vi "vew -- set temperature PID.vi"() -> ()   [LabVIEW 2012]
uses:
  ctl -- name dispatcher -- action.ctl
  tale of three indices.vi
  linear interpolation - real.vi
  line -- complex.vi
  Q -- check range -- i -- integer.vi
  command stack.vi
  tale of three indices -- check state.vi
  Q - not nan -- integer.vi
panel:
  out "df out":dbl
  out "Numeric":i32
  out "Plot: slope 2":cluster{dbl[], dbl[]}[](graph)=[{[], []}, {[10.0, 79.9, 149.8, 219.70000000000002, 289.6, 359.5, 429.40000000000003, 499.30000000000007, 569.2, 639.1, 709.0, 778.9000000000001, 848.8000000000001, 918.7, 988.6000000000001, 1058.5, 1128.4, 1198.3000000000002, 1268.2, 1338.1000000000001, 1408.0, 1477.9, 1547.8000000000002, 1617.7, 1687.6000000000001, 1757.5000000000002, 1827.4, 1897.3000000000002, 1967.2000000000003, 2037.1000000000001, 2107.0, 2176.9, 2246.8, 2316.7000000000003, 2386.6000000000004, 2456.5, 2526.4, 2596.3, 2666.2000000000003, 2736.1000000000004, 2806.0, 2875.9, 2945.8, 3015.7000000000003, 3085.6000000000004, 3155.5000000000005, 3225.4, 3295.3, 3365.2000000000003, 3435.1000000000004, 3505.0000000000005, 3574.9, 3644.8, 3714.7000000000003, 3784.6000000000004, 3854.5000000000005, 3924.4000000000005, 3994.3, 4064.2000000000003, 4134.1, 4204.0, 4273.900000000001, 4343.8, 4413.700000000001, 4483.6, 4553.5, 4623.400000000001, 4693.3, 4763.200000000001, 4833.1, 4903.0, 4972.900000000001, 5042.8, 5112.700000000001, 5182.6, 5252.5, 5322.400000000001, 5392.3, 5462.200000000001, 5532.1, 5602.0, 5671.900000000001, 5741.8, 5811.700000000001, 5881.6, 5951.500000000001, 6021.400000000001, 6091.3, 6161.200000000001, 6231.1, 6301.000000000001, 6370.900000000001, 6440.8, 6510.700000000001, 6580.6, 6650.500000000001, 6720.400000000001, 6790.3, 6860.200000000001, 6930.1], [1.0, 1.0, 1.0, 1.0, 1.0, 1.0, 1.0, 1.0, 1.0, 1.0, 1.0, 1.0, 1.0, 1.0, 1.0, 1.0, 1.0, 1.0, 1.0, 1.0, 1.0, 1.0, 1.0, 1.0, 1.0, 1.0, 1.0, 1.0, 1.0, 1.0, 1.0, 1.0, 1.0, 1.0, 1.0, 1.0, 1.0, 1.0, 1.0, 1.0, 1.0, 1.0, 1.0, 1.0, 1.0, 1.0, 1.0, 1.0, 1.0, 1.0, 1.0, 1.0, 1.0, 1.0, 1.0, 1.0, 1.0, 1.0, 1.0, 1.0, 1.0, 1.0, 1.0, 1.0, 1.0, 1.0, 1.0, 1.0, 1.0, 1.0, 1.0, 1.0, 1.0, 1.0, 1.0, 1.0, 1.0, 1.0, 1.0, 1.0, 1.0, 1.0, 1.0, 1.0, 1.0, 1.0, 1.0, 1.0, 1.0, 1.0, 1.0, 1.0, 1.0, 1.0, 1.0, 1.0, 1.0, 1.0, 1.0, 1.0]}]
  out "Plot: slope":cluster{dbl[], dbl[]}[](graph)=[{[], []}, {[10.0, 79.9, 149.8, 219.70000000000002, 289.6, 359.5, 429.40000000000003, 499.30000000000007, 569.2, 639.1, 709.0, 778.9000000000001, 848.8000000000001, 918.7, 988.6000000000001, 1058.5, 1128.4, 1198.3000000000002, 1268.2, 1338.1000000000001, 1408.0, 1477.9, 1547.8000000000002, 1617.7, 1687.6000000000001, 1757.5000000000002, 1827.4, 1897.3000000000002, 1967.2000000000003, 2037.1000000000001, 2107.0, 2176.9, 2246.8, 2316.7000000000003, 2386.6000000000004, 2456.5, 2526.4, 2596.3, 2666.2000000000003, 2736.1000000000004, 2806.0, 2875.9, 2945.8, 3015.7000000000003, 3085.6000000000004, 3155.5000000000005, 3225.4, 3295.3, 3365.2000000000003, 3435.1000000000004, 3505.0000000000005, 3574.9, 3644.8, 3714.7000000000003, 3784.6000000000004, 3854.5000000000005, 3924.4000000000005, 3994.3, 4064.2000000000003, 4134.1, 4204.0, 4273.900000000001, 4343.8, 4413.700000000001, 4483.6, 4553.5, 4623.400000000001, 4693.3, 4763.200000000001, 4833.1, 4903.0, 4972.900000000001, 5042.8, 5112.700000000001, 5182.6, 5252.5, 5322.400000000001, 5392.3, 5462.200000000001, 5532.1, 5602.0, 5671.900000000001, 5741.8, 5811.700000000001, 5881.6, 5951.500000000001, 6021.400000000001, 6091.3, 6161.200000000001, 6231.1, 6301.000000000001, 6370.900000000001, 6440.8, 6510.700000000001, 6580.6, 6650.500000000001, 6720.400000000001, 6790.3, 6860.200000000001, 6930.1], [1.0, 1.0, 1.0, 1.0, 1.0, 1.0, 1.0, 1.0, 1.0, 1.0, 1.0, 1.0, 1.0, 1.0, 1.0, 1.0, 1.0, 1.0, 1.0, 1.0, 1.0, 1.0, 1.0, 1.0, 1.0, 1.0, 1.0, 1.0, 1.0, 1.0, 1.0, 1.0, 1.0, 1.0, 1.0, 1.0, 1.0, 1.0, 1.0, 1.0, 1.0, 1.0, 1.0, 1.0, 1.0, 1.0, 1.0, 1.0, 1.0, 1.0, 1.0, 1.0, 1.0, 1.0, 1.0, 1.0, 1.0, 1.0, 1.0, 1.0, 1.0, 1.0, 1.0, 1.0, 1.0, 1.0, 1.0, 1.0, 1.0, 1.0, 1.0, 1.0, 1.0, 1.0, 1.0, 1.0, 1.0, 1.0, 1.0, 1.0, 1.0, 1.0, 1.0, 1.0, 1.0, 1.0, 1.0, 1.0, 1.0, 1.0, 1.0, 1.0, 1.0, 1.0, 1.0, 1.0, 1.0, 1.0, 1.0, 1.0]}]
  out "ok":bool
  in  "sweep folder path":path=path "E:/data/Ultrasound/Experiment/ProbeTest/Probe10/YBCO_6/sweep3"
  in  "N":i32=100
  in  "time max":dbl=7000.0
  in  "time min":dbl=10.0
  out "Plot: phase around center":cluster{dbl[], dbl[]}[](graph)=[{[], []}, {[10.0, 79.9, 149.8, 219.70000000000002, 289.6, 359.5, 429.40000000000003, 499.30000000000007, 569.2, 639.1, 709.0, 778.9000000000001, 848.8000000000001, 918.7, 988.6000000000001, 1058.5, 1128.4, 1198.3000000000002, 1268.2, 1338.1000000000001, 1408.0, 1477.9, 1547.8000000000002, 1617.7, 1687.6000000000001, 1757.5000000000002, 1827.4, 1897.3000000000002, 1967.2000000000003, 2037.1000000000001, 2107.0, 2176.9, 2246.8, 2316.7000000000003, 2386.6000000000004, 2456.5, 2526.4, 2596.3, 2666.2000000000003, 2736.1000000000004, 2806.0, 2875.9, 2945.8, 3015.7000000000003, 3085.6000000000004, 3155.5000000000005, 3225.4, 3295.3, 3365.2000000000003, 3435.1000000000004, 3505.0000000000005, 3574.9, 3644.8, 3714.7000000000003, 3784.6000000000004, 3854.5000000000005, 3924.4000000000005, 3994.3, 4064.2000000000003, 4134.1, 4204.0, 4273.900000000001, 4343.8, 4413.700000000001, 4483.6, 4553.5, 4623.400000000001, 4693.3, 4763.200000000001, 4833.1, 4903.0, 4972.900000000001, 5042.8, 5112.700000000001, 5182.6, 5252.5, 5322.400000000001, 5392.3, 5462.200000000001, 5532.1, 5602.0, 5671.900000000001, 5741.8, 5811.700000000001, 5881.6, 5951.500000000001, 6021.400000000001, 6091.3, 6161.200000000001, 6231.1, 6301.000000000001, 6370.900000000001, 6440.8, 6510.700000000001, 6580.6, 6650.500000000001, 6720.400000000001, 6790.3, 6860.200000000001, 6930.1], [1.0, 1.0, 1.0, 1.0, 1.0, 1.0, 1.0, 1.0, 1.0, 1.0, 1.0, 1.0, 1.0, 1.0, 1.0, 1.0, 1.0, 1.0, 1.0, 1.0, 1.0, 1.0, 1.0, 1.0, 1.0, 1.0, 1.0, 1.0, 1.0, 1.0, 1.0, 1.0, 1.0, 1.0, 1.0, 1.0, 1.0, 1.0, 1.0, 1.0, 1.0, 1.0, 1.0, 1.0, 1.0, 1.0, 1.0, 1.0, 1.0, 1.0, 1.0, 1.0, 1.0, 1.0, 1.0, 1.0, 1.0, 1.0, 1.0, 1.0, 1.0, 1.0, 1.0, 1.0, 1.0, 1.0, 1.0, 1.0, 1.0, 1.0, 1.0, 1.0, 1.0, 1.0, 1.0, 1.0, 1.0, 1.0, 1.0, 1.0, 1.0, 1.0, 1.0, 1.0, 1.0, 1.0, 1.0, 1.0, 1.0, 1.0, 1.0, 1.0, 1.0, 1.0, 1.0, 1.0, 1.0, 1.0, 1.0, 1.0]}]
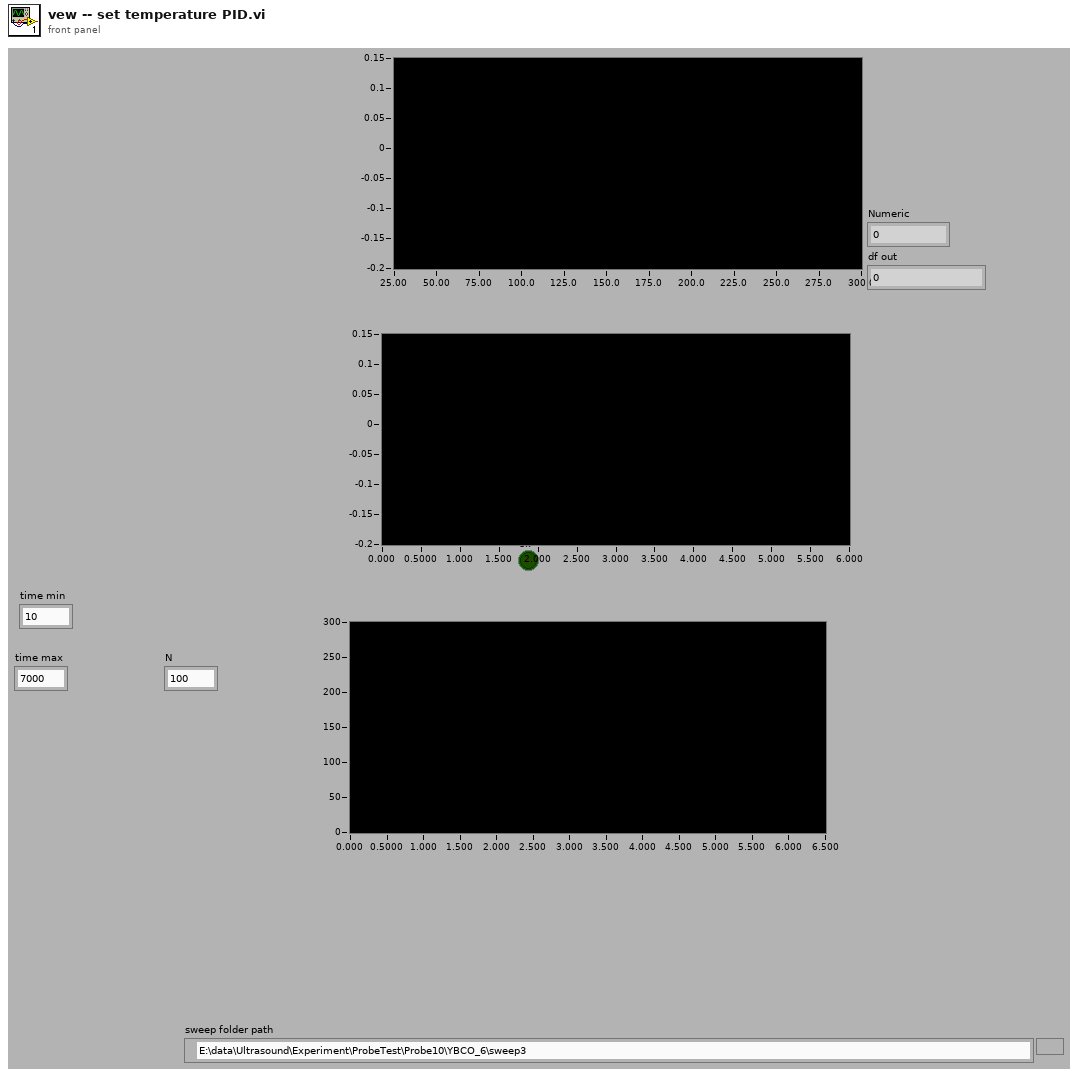
[diagram p1: front panel]
types:
  T1 = typedef "ctl -- name dispatcher -- action.ctl" = enum16{"peak frequency", "peak frequency DUMP", "peak gamma DUMP", "peak gamma", "peak frequency TEST", "peak gamma TEST", "power", "time in gamma", "set temperature ", "set temperature timer", "peak default gamma", "last scan file", "peak freq gamma TEST", "peak NAMES"}
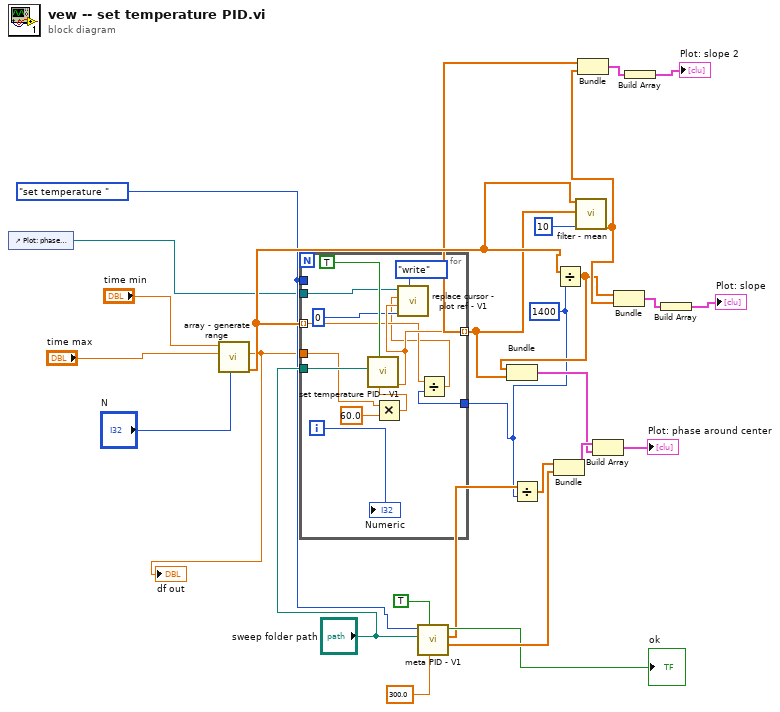
[diagram p0: block diagram]
diagram:
  w4 = ctl_--_name_dispatcher_--_action."set temperature " ("ctl name dispatch")
  w1 = 1400 ("window")
  n1 = control-ref of="Plot: phase around center"() -> (w2:refnum<vi>)
  n2 = call "array - generate range.vi"("N"="N", "freq max"="time max", "freq min"="time min") -> ("Array"=w12:dbl[], "df out"=w3:dbl)  [unwired: 7 in]
  "df out" <- w3
  n3 = for {
    tunnel: w12 -> [w29] mode=indexing
    tunnel: [w32] -> w9 mode=indexing
    tunnel: "sweep folder path" -> [w39]
    tunnel: w4 -> [_]
    tunnel: w3 -> [w36]
    tunnel: w2 -> [w34]
    tunnel: w1 -> [w30]
    i -> [w27]
    n4 = Multiply(x=w36, y=60.0) -> (x*y=w35:dbl)
    n5 = call "set temperature PID - V1.vi"("delta time(sec)"=w35, "control set temperature PID?"=TRUE ("control power PID?"), "sweep folder path"=w39) -> ("next set temperature"=w32:dbl)  [unwired: 6 in, 2 out]
    n6 = Divide(x=w29, y=w30) -> (x/y=w28:dbl)
    n7 = call "replace cursor - plot ref - V1.vi"("action"=enum16{"", "read", "write"}."write", "cursor index"=0, "new  Y"=w32, "new X"=w28, "Plot ref in"=w34) -> ()  [unwired: 4 in, 3 out]
    "Numeric" <- w27
  }
  n8 = call "meta PID - V1.vi"("current temperature"=300.0 ("nonzero temperature"), "control power PID?"=TRUE, "sweep folder path"="sweep folder path", "ctl name dispatch"=w4) -> ("frequencies"=w20:dbl[], "temperatures"=w6:dbl[], "ok"=→"ok":bool)  [unwired: 4 in, 1 out]
  n9 = Divide(x=w6, y=w1) -> (x/y=w5:dbl[])
  n10 = Bundle(w5, "frequencies"=w20) -> (w26:cluster{dbl[], "frequencies":dbl[]})  [unwired: 1 in]
  n11 = Divide(x=w12, y=w1) -> (x/y=w7:dbl[])
  n12 = Bundle(w7, w9) -> (w22:cluster{dbl[], dbl[]})  [unwired: 1 in]
  n13 = call "filter - mean.vi"("omega  in"=w12, "z in"=w9, "window"=10) -> ("slope"=w8:dbl[])  [unwired: 13 in, 3 out]
  n14 = Bundle(w9, "slope"=w8) -> (w11:cluster{dbl[], "slope":dbl[]})  [unwired: 1 in]
  n15 = Build Array(w26, w22) -> (→"Plot: phase around center":cluster{dbl[], "frequencies":dbl[]}[])
  n16 = Bundle(w7, "slope"=w8) -> (w15:cluster{dbl[], "slope":dbl[]})  [unwired: 1 in]
  n17 = Build Array(w11) -> (→"Plot: slope 2":cluster{dbl[], "slope":dbl[]}[])
  n18 = Build Array(w15) -> (→"Plot: slope":cluster{dbl[], "slope":dbl[]}[])
